vi "計算式.vi"(0 "b y":i32, 5 "投彈時間(k)":dbl, 7 "Va":dbl, 9 "Vc":dbl, 11 "S0":i32, 12 "H":dbl, 13 "stop":bool, 14 "ti":dbl) -> (4 "b y 2":dbl, 6 "output stop":bool, 8 "a x":dbl, 10 "c x":dbl, 15 "to":dbl)   [LabVIEW 2014]
panel:
  out "投彈時間(k)":dbl
  in  "S0":i32=630
  in  "Vc":dbl=30.0
  in  "Va":dbl=120.0
  in  "H":dbl=122.5
  in  "stop":bool
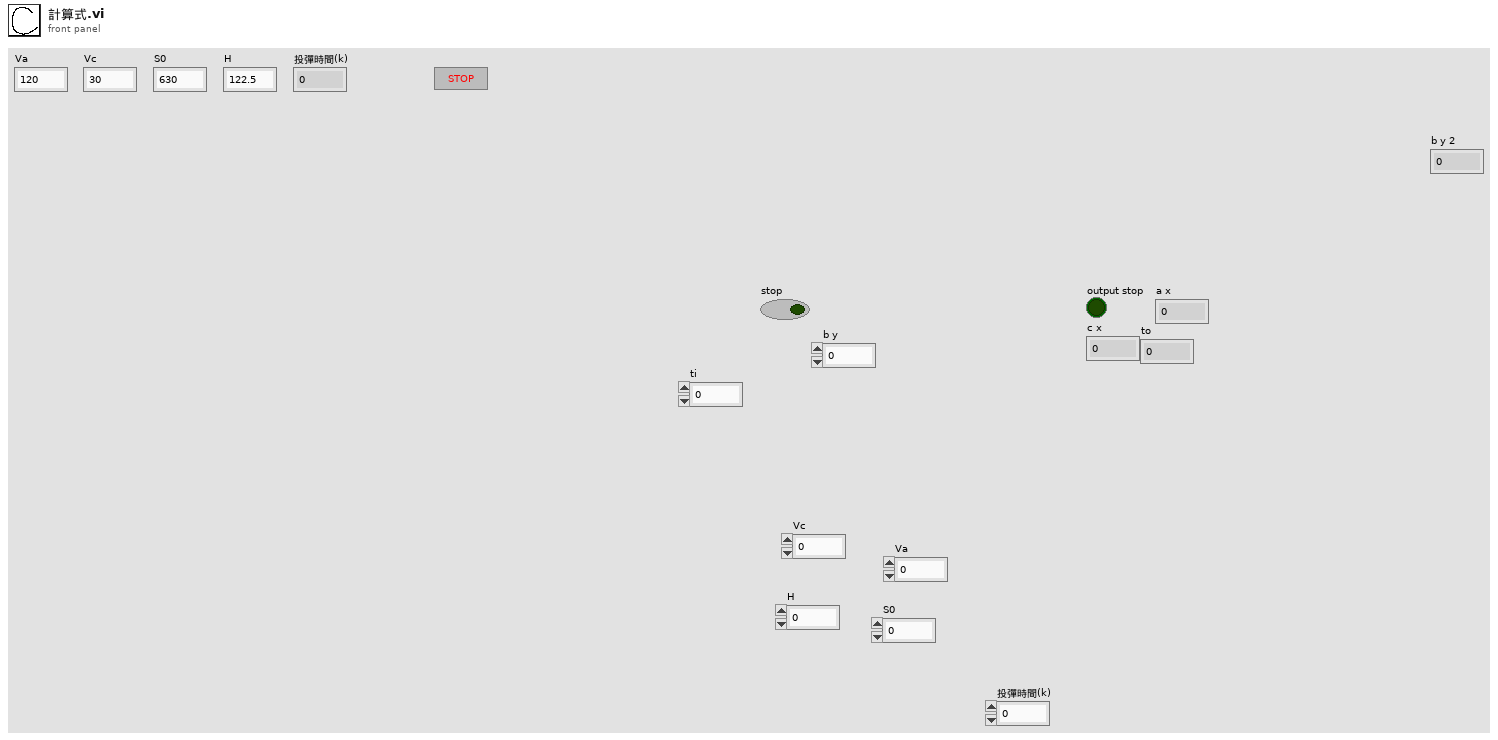
[diagram p1: front panel]
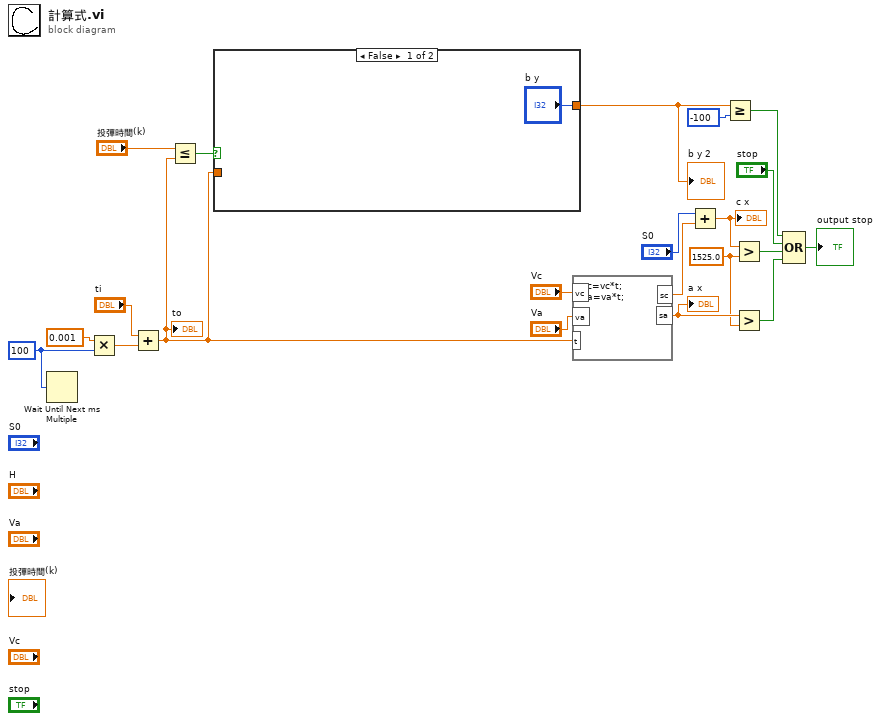
[diagram p0: block diagram]
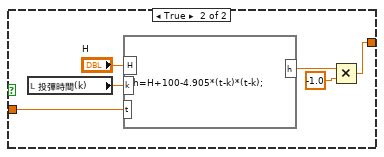
[diagram p2: hidden frame]
diagram:
  w2 = 1525.0 ("y")
  w21 = u32 100
  n1 = Wait Until Next ms Multiple(millisecond multiple=w21) -> ()  [unwired: 1 out]
  n2 = Multiply(x=0.001, y=w21) -> (x*y=w20:dbl)
  n3 = Add(x="ti", y=w20) -> (x+y=w14:dbl)
  "to" <- w14
  n4 = Less Or Equal?(x="投彈時間(k)", y=w14) -> (x <= y?=w19:bool)
  n5 = case shown="False" w19 {
    tunnel: ["b y" w27] -> w17
    tunnel: w14 -> [_ w26]
    frame False {
    }
    frame True {
      n6 = local read "投彈時間(k)"() -> (w24:dbl)
      n7 = formula code="h=H+100-4.905*(t-k)*(t-k);"("H"="H", "t"=w26, "k"=w24) -> ("h"=w28:dbl)
      n8 = Multiply(x=w28, y=-1.0) -> (x*y=w27:dbl)
    }
  }
  "b y 2" <- w17
  n9 = formula code="sc=vc*t;\nsa=va*t;"("vc"="Vc", "t"=w14, "va"="Va") -> ("sc"=w15:dbl, "sa"=w3:dbl)
  "a x" <- w3
  n10 = Add(x="S0", y=w15) -> (x+y=w8:dbl)
  "c x" <- w8
  n11 = Greater Or Equal?(x=w17, y=-100) -> (x >= y?=w7:bool)
  n12 = Greater?(x=w8, y=w2) -> (0:w5:bool)
  n13 = Greater?(x=w3, y=w2) -> (0:w1:bool)
  n14 = Compound Arithmetic op=OR(w7, "stop", w5, w1) -> (→"output stop":bool)
